vi "ListAttributes.vi"(6 "Inheritable Only? (F: all)":bool, 8 "error in (no error)":errorcluster, 11 "SMO in":refnum<class "SMO.lvclass">) -> (0 "error out":errorcluster, 2 "[Attributes]":refnum<class "Attribute.lvclass">[](array[class]), 3 "SMO out":refnum<class "SMO.lvclass">)   [LabVIEW 2019, in "SMO.lvclass"]
doc: "JKI State Machine Objects (SMO) 1.3.0.56\nJKI - JKI\nCopyright (c) 2017, JKI"
uses:
  SMO.lvclass
  Support/Attribute/Attribute.lvclass
  SMO.lvclass/SMO.ctl
  Support/Attribute/Attribute.lvclass/Attribute.ctl
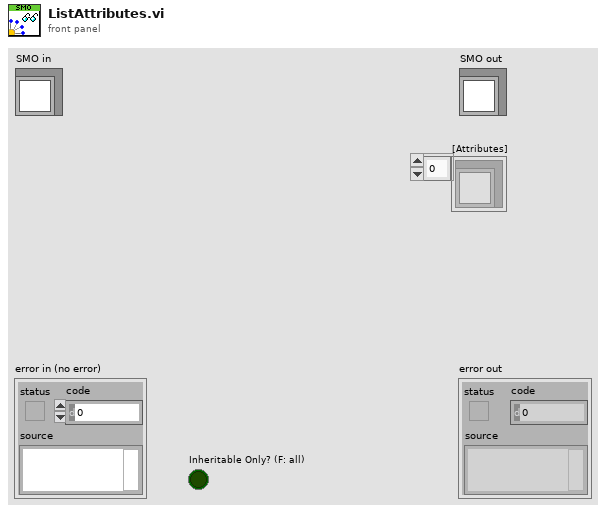
[diagram p1: front panel]
types:
  T1 = typedef "SMO.lvclass/PrivateData--Ref.ctl" = refnum<data-value>
  T2 = typedef "SMO.lvclass/PrivateData--Cluster.ctl" = cluster{"Parent Call":T3, "Registered Processes":T4[], "Sync Notifier":refnum<notifier>, "Process Error Notifier":refnum<notifier>, "Protected Events":T5, "Public Events":T6, "SMO State":T7, "[Dependencies]":T8[], "[Attributes]":refnum<class "Attribute.lvclass">[], "Launcher Close":refnum<notifier>, "Caller Watchdog":refnum<queue>, "Accessibility":T9, "NbStaticDependencies":u32}
  T3 = typedef "SMO.lvclass/Parent Call--Enum.ctl" = enum16{"Allows parent to run", "Does not request parent to run"}
  T4 = typedef "SMO.lvclass/RegisteredProcessData--Cluster.ctl" = cluster{"Name":string, "Static VI Ref":refnum<vi>, "Running":bool, "NotifierRef":u32}
  T5 = typedef "SMO.lvclass/Protected Events.ctl" = cluster{"StopProcesses":refnum<user-event>, "AbortProcesses":refnum<user-event>, "Config Changed":refnum<user-event>, "Dependency":refnum<user-event>}
  T6 = typedef "SMO.lvclass/Public Events.ctl" = cluster{"Error":refnum<user-event>, "State":refnum<user-event>, "Reserve State":refnum<user-event>}
  T7 = typedef "SMO.lvclass/SMOState --Enum.ctl" = enum16{"unknown", "Created", "Started", "Stopped"}
  T8 = typedef "SMO.lvclass/SMO Dependency--Cluster.ctl" = cluster{"Dependency":refnum<class "SMO.lvclass">, "Level":string}
  T9 = typedef "SMO.lvclass/Accessibility--Cluster.ctl" = cluster{"Lock Key":string, "Reserve State":T10}
  T10 = typedef "SMO.lvclass/Reserve State--Enum.ctl" = enum16{"Unreserved", "Reserved", "Self-locked"}
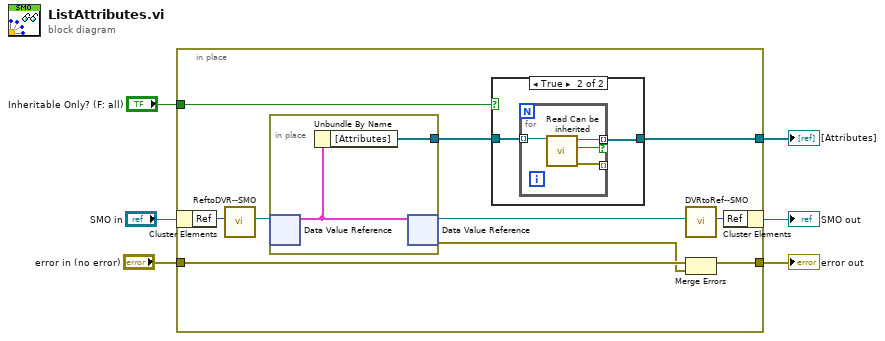
[diagram p0: block diagram]
diagram:
  n1 = in-place {
    in-place-border: "error in (no error)" -> [w12]
    in-place-border: [w10] -> w3
    in-place-border: [w7] -> w2
    in-place-border: "Inheritable Only? (F: all)" -> [w9]
    n2 = in-place-cluster #1("SMO in") -> ("Ref"=w16:u32)
    n3 = call "ReftoDVR--SMO.vi"("Ref"=w16) -> ("Ref"=w15:T1)  [unwired: 10 in]
    n4 = in-place {
      in-place-border: [w24] -> w8
      n5 = in-place-dvr #2(w15) -> (w25:T2)  [unwired: 1 out]
      n6 = Unbundle By Name(w25) -> ("[Attributes]"=w24:refnum<class "Attribute.lvclass">[])
      n7 = in-place-dvr #2(w25) -> (w14:T1, w11:errorcluster)
    }
    n8 = case shown="True" w9 {
      tunnel: w8 -> [w17 w19]
      tunnel: [w17 w18] -> w7
      frame False {
      }
      frame True {
        n9 = for {
          tunnel: w19 -> [w23] mode=indexing
          tunnel: [w22] -> w18 mode=indexing if=w21
          tunnel: [w20] -> _ mode=indexing
          n10 = call "Read Can be inherited.vi"("Attribute in"=w23) -> ("error out"=w20:errorcluster, "Can be inherited"=w21:bool, "Attribute out"=w22:refnum<class "Attribute.lvclass">)  [unwired: 8 in]
        }
      }
    }
    n11 = call "DVRtoRef--SMO.vi"("Ref"=w14) -> ("Ref"=w13:u32)  [unwired: 10 in]
    n12 = Merge Errors(w12, w11) -> (w10:errorcluster)
    n13 = in-place-cluster #1("Ref"=w13) -> (→"SMO out":refnum<class "SMO.lvclass">)
  }
  "error out" <- w3
  "[Attributes]" <- w2
